vi "ADIS16448 CRC.vi"(7 "Look-Up Table Method?":bool, 10 "Byte Array (MSB-First)":u8[](array[numeric])) -> (2 "CRC16-ADIS":u16)   [LabVIEW 2019]
panel:
  # "This vi calculates a CRC16 check on data generated from an \nADIS16448 IMU when using burst mode (MSC_CTRL[4] = 1). \nThis implementation is a variant of the CCITT X.25 spec.\n\nJuan Chong - December 2017"
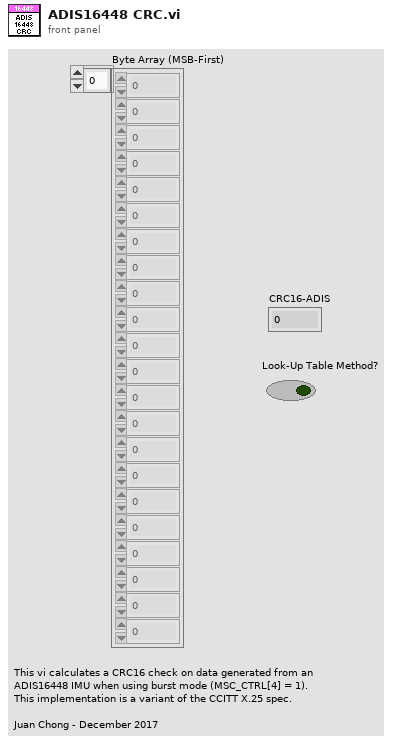
[diagram p1: front panel]
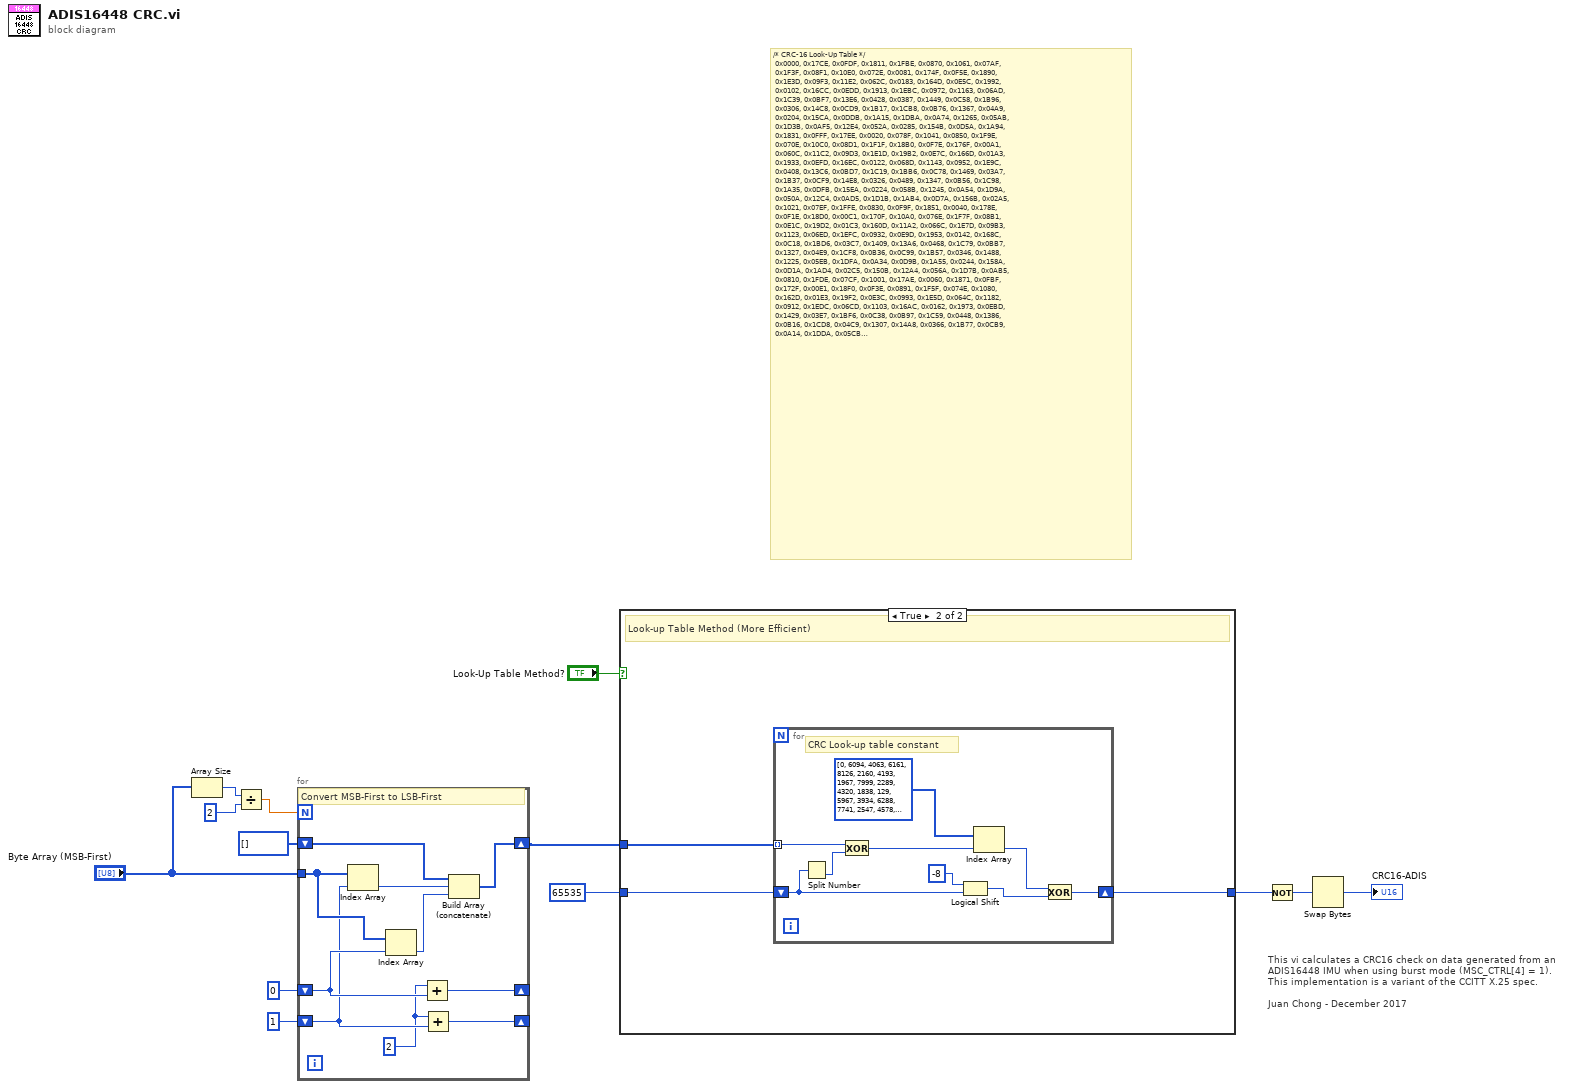
[diagram p0: block diagram]
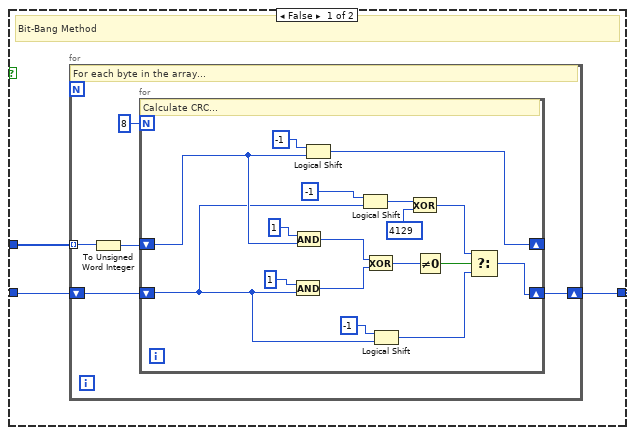
[diagram p2: hidden frame]
diagram:
  # "/* CRC-16 Look-Up Table */\n\t0x0000, 0x17CE, 0x0FDF, 0x1811, 0x1FBE, 0x0870, 0x1061, 0x07AF,\n\t0x1F3F, 0x08F1, 0x10E0, 0x072E, 0x0081, 0x174F, 0x0F5E, 0x1890,\n\t0x1E3D, 0x09F3, 0x11E2, 0x062C, 0x0183, 0x164D, 0x0E5C, 0x1992,\n\t0x0102, 0x16CC, 0x0EDD, 0x1913, 0x1EBC, 0x0972, 0x1163, 0x06AD,\n\t0x1C39, 0x0BF7, 0x13E6, 0x0428, 0x0387, 0x1449, 0x0C58, 0x1B96,\n\t0x0306, 0x14C8, 0x0CD9, 0x1B17, 0x1CB8, 0x0B76, 0x1367, 0x04A9,\n\t0x0204, 0x15CA, 0x0DDB, 0x1A15, 0x1DBA, 0x0A74, 0x1265, 0x05AB,\n\t0x1D3B, 0x0AF5, 0x12E4, 0x052A, 0x0285, 0x154B, 0x0D5A, 0x1A94,\n\t0x1831, 0x0FFF, 0x17EE, 0x0020, 0x078F, 0x1041, 0x0850, 0x1F9E,\n\t0x070E, 0x10C0, 0x08D1, 0x1F1F, 0x18B0, 0x0F7E, 0x176F, 0x00A1,\n\t0x060C, 0x11C2, 0x09D3, 0x1E1D, 0x19B2, 0x0E7C, 0x166D, 0x01A3,\n\t0x1933, 0x0EFD, 0x16EC, 0x0122, 0x068D, 0x1143, 0x0952, 0x1E9C,\n\t0x0408, 0x13C6, 0x0BD7, 0x1C19, 0x1BB6, 0x0C78, 0x1469, 0x03A7,\n\t0x1B37, 0x0CF9, 0x14E8, 0x0326, 0x0489, 0x1347, 0x0B56, 0x1C98,\n\t0x1A35, 0x0DFB, 0x15EA, 0x0224, 0x058B, 0x1245, 0x0A54, 0x1D9A,\n\t0x050A, 0x12C4, 0x0AD5, 0x1D1B, 0x1AB4, 0x0D7A, 0x156B, 0x02A5,\n\t0x1021, 0x07EF, 0x1FFE, 0x0830, 0x0F9F, 0x1851, 0x0040, 0x178E,\n\t0x0F1E, 0x18D0, 0x00C1, 0x170F, 0x10A0, 0x076E, 0x1F7F, 0x08B1,\n\t0x0E1C, 0x19D2, 0x01C3, 0x160D, 0x11A2, 0x066C, 0x1E7D, 0x09B3,\n\t0x1123, 0x06ED, 0x1EFC, 0x0932, 0x0E9D, 0x1953, 0x0142, 0x168C,\n\t0x0C18, 0x1BD6, 0x03C7, 0x1409, 0x13A6, 0x0468, 0x1C79, 0x0BB7,\n\t0x1327, 0x04E9, 0x1CF8, 0x0B36, 0x0C99, 0x1B57, 0x0346, 0x1488,\n\t0x1225, 0x05EB, 0x1DFA, 0x0A34, 0x0D9B, 0x1A55, 0x0244, 0x158A,\n\t0x0D1A, 0x1AD4, 0x02C5, 0x150B, 0x12A4, 0x056A, 0x1D7B, 0x0AB5,\n\t0x0810, 0x1FDE, 0x07CF, 0x1001, 0x17AE, 0x0060, 0x1871, 0x0FBF,\n\t0x172F, 0x00E1, 0x18F0, 0x0F3E, 0x0891, 0x1F5F, 0x074E, 0x1080,\n\t0x162D, 0x01E3, 0x19F2, 0x0E3C, 0x0993, 0x1E5D, 0x064C, 0x1182,\n\t0x0912, 0x1EDC, 0x06CD, 0x1103, 0x16AC, 0x0162, 0x1973, 0x0EBD,\n\t0x1429, 0x03E7, 0x1BF6, 0x0C38, 0x0B97, 0x1C59, 0x0448, 0x1386,\n\t0x0B16, 0x1CD8, 0x04C9, 0x1307, 0x14A8, 0x0366, 0x1B77, 0x0CB9,\n\t0x0A14, 0x1DDA, 0x05CB, 0x1205, 0x15AA, 0x0264, 0x1A75, 0x0DBB,\n\t0x152B, 0x02E5, 0x1AF4, 0x0D3A, 0x0A95, 0x1D5B, 0x054A, 0x1284"
  # "This vi calculates a CRC16 check on data generated from an \nADIS16448 IMU when using burst mode (MSC_CTRL[4] = 1). \nThis implementation is a variant of the CCITT X.25 spec.\n\nJuan Chong - December 2017"
  n1 = Array Size(array="Byte Array (MSB-First)") -> (size(s)=w4:i32)
  n2 = Divide(x=w4, y=2) -> (x/y=w3:dbl)
  n3 = for {
    N: w3 -> [_]
    tunnel: "Byte Array (MSB-First)" -> [w23]
    shift-right: [w20] -> _
    shift-left: 0 -> [w22]
    shift-right: [w21] -> _
    shift-left: 1 -> [w19]
    shift-right: [w15] -> w2
    shift-left: u8[] [] -> [w14]
    w18 = 2 ("x")
    # "Convert MSB-First to LSB-First"
    n4 = Index Array(array=w23, index=w19) -> (element=w17:u8)
    n5 = Index Array(array=w23, index=w22) -> (element=w16:u8)
    n6 = Add(x=w18, y=w22) -> (x+y=w20:i32)
    n7 = Add(x=w18, y=w19) -> (x+y=w21:i32)
    n8 = Build Array (concatenate)(w14, w17, w16) -> (w15:u8[])
  }
  n9 = case shown="True" "Look-Up Table Method?" {
    tunnel: w2 -> [w26 w51]
    tunnel: [w25 w50] -> w13
    tunnel: u16 65535 -> [w24 w49]
    frame False {
      # "Bit-Bang Method"
      n10 = for {
        tunnel: w26 -> [w28] mode=indexing
        shift-right: [w30] -> w25
        shift-left: w24 -> [w31]
        # "For each byte in the array..."
        n11 = To Unsigned Word Integer(number=w28) -> (unsigned 16bit integer=w27:u16)
        n12 = for {
          N: 8 -> [_]
          shift-right: [w38] -> w30
          shift-left: w31 -> [w32]
          shift-right: [w34] -> _
          shift-left: w27 -> [w33]
          # "Calculate CRC..."
          n13 = And(x=u16 1, y=w32) -> (x .and. y?=w47:u16)
          n14 = And(x=u16 1, y=w33) -> (x .and. y?=w36:u16)
          n15 = Logical Shift(y=i16 -1, x=w33) -> (x << y=w34:u16)
          n16 = Logical Shift(y=i16 -1, x=w32) -> (x << y=w43:u16)
          n17 = Exclusive Or(1:w47, 2:w36) -> (0:w46:u16)
          n18 = Logical Shift(y=i16 -1, x=w32) -> (x << y=w39:u16)
          n19 = Exclusive Or(1:u16 4129, 2:w43) -> (0:w41:u16)
          n20 = Not Equal To 0?(x=w46) -> (x != 0?=w45:bool)
          n21 = Select(t=w41, s=w45, f=w39) -> (s? t:f=w38:u16)
        }
      }
    }
    frame True {
      # "Look-up Table Method (More Efficient)"
      n22 = for {
        tunnel: w51 -> [w54] mode=indexing
        shift-right: [w58] -> w50
        shift-left: w49 -> [w56]
        # "CRC Look-up table constant"
        n23 = Split Number(x=w56) -> (lo(x)=w55:u8)  [unwired: 1 out]
        n24 = Exclusive Or(1:w55, 2:w54) -> (0:w53:u8)
        n25 = Logical Shift(y=i8 -8, x=w56) -> (x << y=w59:u16)
        n26 = Index Array(array=u16[] [0, 6094, 4063, 6161, 8126, 2160, 4193, 1967, 7999, 2289, 4320, 1838, 129, 5967, 3934, 6288, 7741, 2547, 4578, 1580, 387, 5709, 3676, 6546, 258, 5836, 3805, 6419, 7868, 2418, 4451, 1709, 7225, 3063, 5094, 1064, 903, 5193, 3160, 7062, 774, 5320, 3289, 6935, 7352, 2934, 4967, 1193, 516, 5578, 3547, 6677, 7610, 2676, 4709, 1451, 7483, 2805, 4836, 1322, 645, 5451, 3418, 6804, 6193, 4095, 6126, 32, 1935, 4161, 2128, 8094, 1806, 4288, 2257, 7967, 6320, 3966, 5999, 161, 1548, 4546, 2515, 7709, 6578, 3708, 5741, 419, 6451, 3837, 5868, 290, 1677, 4419, 2386, 7836, 1032, 5062, 3031, 7193, 7094, 3192, 5225, 935, 6967, 3321, 5352, 806, 1161, 4935, 2902, 7320, 6709, 3579, 5610, 548, 1419, 4677, 2644, 7578, 1290, 4804, 2773, 7451, 6836, 3450, 5483, 677, 4129, 2031, 8190, 2096, 3999, 6225, 64, 6030, 3870, 6352, 193, 5903, 4256, 1902, 8063, 2225, 3612, 6610, 451, 5645, 4514, 1644, 7805, 2483, 4387, 1773, 7932, 2354, 3741, 6483, 322, 5772, 3096, 7126, 967, 5129, 5030, 1128, 7289, 2999, 4903, 1257, 7416, 2870, 3225, 6999, 838, 5256, 4645, 1515, 7674, 2612, 3483, 6741, 580, 5514, 3354, 6868, 709, 5387, 4772, 1386, 7547, 2741, 2064, 8158, 1999, 4097, 6062, 96, 6257, 4031, 5935, 225, 6384, 3902, 2193, 8031, 1870, 4224, 5677, 483, 6642, 3644, 2451, 7773, 1612, 4482, 2322, 7900, 1741, 4355, 5804, 354, 6515, 3773, 5161, 999, 7158, 3128, 2967, 7257, 1096, 4998, 2838, 7384, 1225, 4871, 5288, 870, 7031, 3257, 2580, 7642, 1483, 4613, 5546, 612, 6773, 3515, 5419, 741, 6900, 3386, 2709, 7515, 1354, 4740] ("CRC-16 Lookup Table 2"), index=w53) -> (element=w57:u16)
        n27 = Exclusive Or(1:w59, 2:w57) -> (0:w58:u16)
      }
    }
  }
  n28 = Not(x=w13) -> (.not. x?=w12:u16)
  n29 = Swap Bytes(anything=w12) -> (byte swapped=→"CRC16-ADIS":u16)
